vi "OrderParams.vi"(6 "UseLV2011Compatability":bool, 7 "Terminal Bounds[]":T2[](array[typedef]), 8 "Param Names":string[](array[string]), 9 "Data types":string[](array[string]), 10 "Dirs":T1[](array[typedef]), 11 "Connum":i32[](array[numeric])) -> (0 "Param Names out":string[](array[string]), 1 "Data types  out":string[](array[string]), 2 "Dirs Out":T1[](array[typedef]), 3 "Connum out":i32[](array[numeric]))   [LabVIEW 2020]
uses:
  <vilib>/AppBuilder/IOStatus.ctl
  <vilib>/Utility/miscctls.llb/LVRectTypeDef.ctl
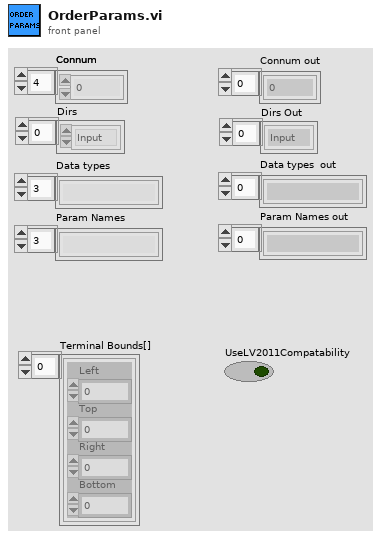
[diagram p1: front panel]
types:
  T1 = typedef "IOStatus.ctl" = enum16{"Input", "Output", "Input/Output", "InputDeleted", "OutputDeleted", "IODeleted", "ErrorClusterIn", "ErrorClusterOut"}
  T2 = typedef "LVRectTypeDef.ctl" = cluster{"Left":i16, "Top":i16, "Right":i16, "Bottom":i16}
  T3 = cluster{"dir":T1, "Left":i16, "Top":i16, "Connum":i32, "Data types":string, "Param Names":string}
  T4 = cluster{"dir":T1, "Left":i16, "Top":i16, "Connum":i32, "Data types":string, "Param Names":string}[]
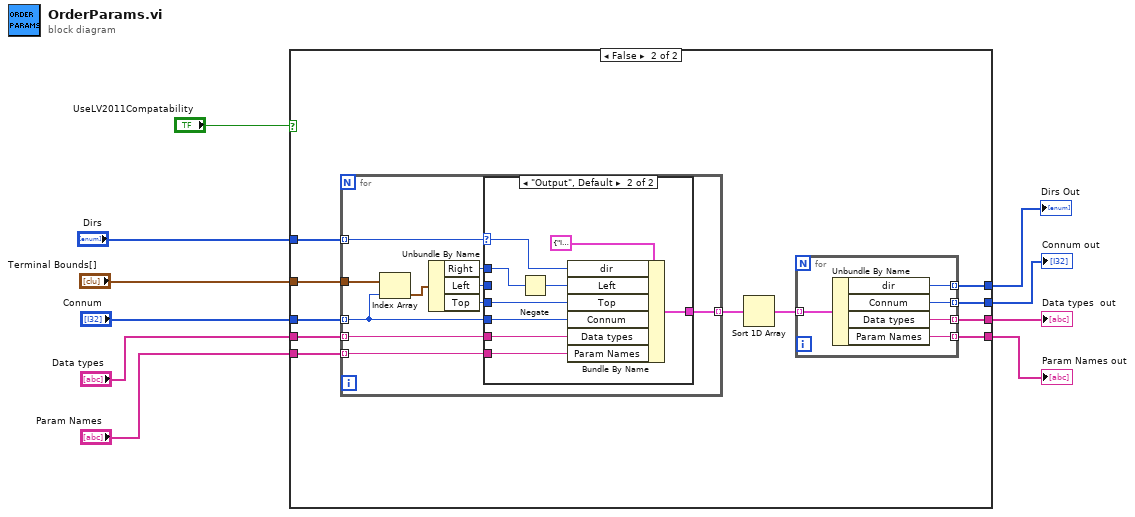
[diagram p0: block diagram]
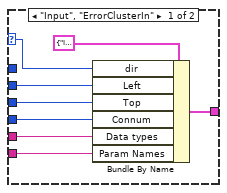
[diagram p3: hidden frame]
diagram:
  n1 = case shown="False" "UseLV2011Compatability" {
    tunnel: "Terminal Bounds[]" -> [_ w23]
    tunnel: [w13 w22] -> w9
    tunnel: [w12 w21] -> w8
    tunnel: [w11 w20] -> w7
    tunnel: "Connum" -> [w13 w19]
    tunnel: "Data types" -> [w12 w18]
    tunnel: "Param Names" -> [w11 w17]
    tunnel: "Dirs" -> [w14 w16]
    tunnel: [w14 w15] -> w4
    frame True {
    }
    frame False {
      n2 = for {
        tunnel: w23 -> [w40]
        tunnel: [w36] -> w24 mode=indexing
        tunnel: w16 -> [w32] mode=indexing
        tunnel: w19 -> [w35] mode=indexing
        tunnel: w18 -> [w34] mode=indexing
        tunnel: w17 -> [w33] mode=indexing
        n3 = Index Array(array=w40, index=w35) -> (element=w39:T2)
        n4 = Unbundle By Name(w39) -> ("Right"=w31:i16, "Left"=w38:i16, "Top"=w37:i16)
        n5 = case shown="\"Output\", Default" w32 {
          selector: w32 -> [w41 w50]
          tunnel: w35 -> [w45 w56]
          tunnel: w38 -> [w47 _]
          tunnel: w37 -> [w46 w57]
          tunnel: w34 -> [w44 w55]
          tunnel: w33 -> [w43 w54]
          tunnel: [w42 w51] -> w36
          tunnel: w31 -> [_ w49]
          frame "Input", "ErrorClusterIn" {
            n6 = Bundle By Name(cluster=T3 {"dir"=enum."Input", "Left"=0, "Top"=0, "Connum"=0, "Data types"="", "Param Names"=""} ("output cluster"), "dir"=w41, "Left"=w47, "Top"=w46, "Connum"=w45, "Data types"=w44, "Param Names"=w43) -> (w42:T3)
          }
          frame "Output", Default {
            n7 = Negate(x=w49) -> (-x=w53:i16)
            n8 = Bundle By Name(cluster=T3 {"dir"=enum."Input", "Left"=0, "Top"=0, "Connum"=0, "Data types"="", "Param Names"=""} ("output cluster"), "dir"=w50, "Left"=w53, "Top"=w57, "Connum"=w56, "Data types"=w55, "Param Names"=w54) -> (w51:T3)
          }
        }
      }
      n9 = Sort 1D Array(array=w24) -> (sorted array=w25:T4)
      n10 = for {
        tunnel: w25 -> [w30] mode=indexing
        tunnel: [w29] -> w15 mode=indexing
        tunnel: [w28] -> w22 mode=indexing
        tunnel: [w27] -> w21 mode=indexing
        tunnel: [w26] -> w20 mode=indexing
        n11 = Unbundle By Name(w30) -> ("dir"=w29:T1, "Connum"=w28:i32, "Data types"=w27:string, "Param Names"=w26:string)
      }
    }
  }
  "Data types  out" <- w8
  "Param Names out" <- w7
  "Connum out" <- w9
  "Dirs Out" <- w4
